vi "TDC_createHbtFunction.vi"(8 "Error In":errorcluster) -> (0 "Error Out":errorcluster, 3 "Function":u64)   [LabVIEW 2011]
uses:
  tdcbase.dll
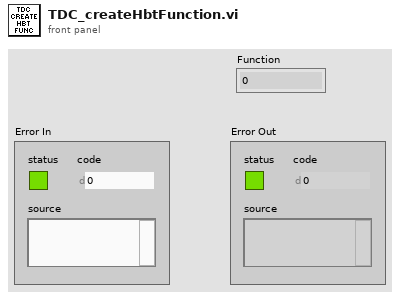
[diagram p1: front panel]
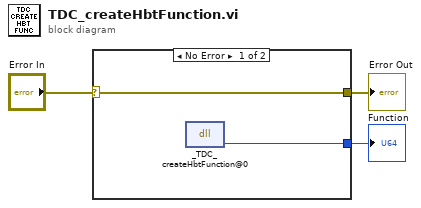
[diagram p0: block diagram]
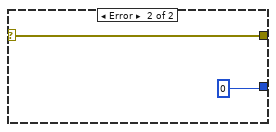
[diagram p2: hidden frame]
diagram:
  n1 = case shown="No Error" "Error In" {
    selector: "Error In" -> [w5 w7]
    tunnel: [w5 w7] -> w2
    tunnel: [w4 u64 0] -> w1
    frame No Error {
      n2 = dll-call lib="X:/tdcbase.dll" fn="_TDC_createHbtFunction@0"() -> ("return type"=w4:u64)  [unwired: 3 in, 2 out]
    }
    frame Error {
    }
  }
  "Error Out" <- w2
  "Function" <- w1
